vi "temp_selection_saving.vi"(8 "error in (no error)":errorcluster, 9 "temp selection":string, 10 "Enum":enum16{"Write", "Read Values"}(ring), 11 "configuration file path":path) -> (0 "error out":errorcluster, 2 "selection_temp":string, 3 "file path":path)   [LabVIEW 2021]
uses:
  <vilib>/Utility/config.llb/Write Key (String).vi
  <vilib>/Utility/config.llb/Read Key (String).vi
  <vilib>/Utility/config.llb/NI_LVConfig.lvlib
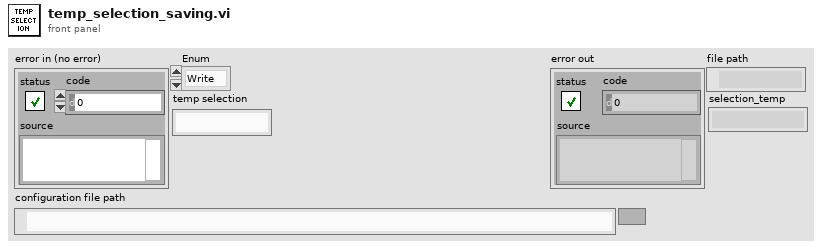
[diagram p1: front panel]
types:
  T1 = typedef "NI_LVConfig.lvlib/Config Data RefNum.ctl" = refnum<k1>
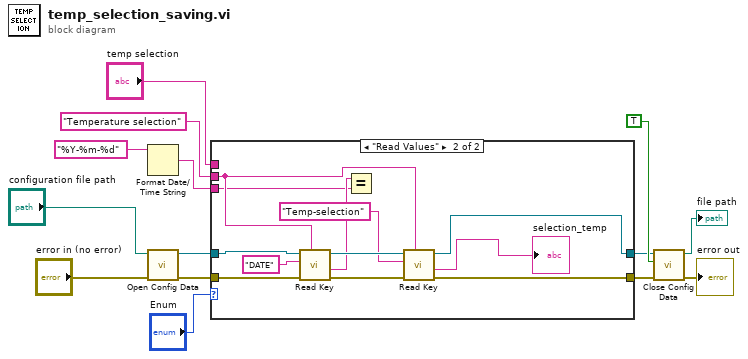
[diagram p0: block diagram]
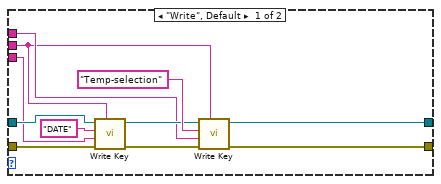
[diagram p2: hidden frame]
diagram:
  n1 = Format Date/Time String(time format string (%c)="%Y-%m-%d") -> (date/time string=w2:string)  [unwired: 2 in]
  n2 = call <vilib>:"Open Config Data.vi"("error in (no error)"="error in (no error)", "configuration file path"="configuration file path") -> ("error out"=w10:errorcluster, "refnum"=w9:T1)  [unwired: 7 in, 1 out]
  n3 = case shown="\"Read Values\"" "Enum" {
    tunnel: w10 -> [w19 w33]
    tunnel: w9 -> [w18 w32]
    tunnel: [w24 w31] -> w6
    tunnel: [w23 w30] -> w7
    tunnel: "Temperature selection" ("String") -> [w15 w34]
    tunnel: w2 -> [w16 w27]
    tunnel: "temp selection" -> [w17 _]
    frame "Write", Default {
      n4 = call-poly <vilib>:"Write Key.vi"("section"=w15, "error in (no error)"=w19, "value"=w16, "key"="DATE", "refnum"=w18) -> ("error out"=w20:errorcluster, "refnum out"=w21:T1)  [unwired: 4 in, 1 out]
      n5 = call-poly <vilib>:"Write Key.vi"("section"=w15, "error in (no error)"=w20, "value"=w17, "key"="Temp-selection", "refnum"=w21) -> ("error out"=w23:errorcluster, "refnum out"=w24:T1)  [unwired: 4 in, 1 out]
    }
    frame "Read Values" {
      n6 = call-poly <vilib>:"Read Key.vi"("section"=w34, "error in (no error)"=w33, "key"="DATE", "refnum"=w32) -> ("error out"=w35:errorcluster, "value"=w28:string, "refnum out"=w36:T1)  [unwired: 4 in, 1 out]
      n7 = Equal?(x=w28, y=w27) -> ()  [unwired: 1 out]
      n8 = call-poly <vilib>:"Read Key.vi"("section"=w34, "error in (no error)"=w35, "key"="Temp-selection", "refnum"=w36) -> ("error out"=w30:errorcluster, "value"=→"selection_temp":string, "refnum out"=w31:T1)  [unwired: 4 in, 1 out]
    }
  }
  n9 = call <vilib>:"Close Config Data.vi"("error in (no error)"=w7, "write file if changed (T)"=TRUE, "refnum"=w6) -> ("error out"=→"error out":errorcluster, "file path"=→"file path":path)  [unwired: 7 in]
